vi "Servo.vi"() -> ()   [LabVIEW 2013]
doc: "This example shows how to set and read the angle of a servo."
uses:
  <vilib>/Rock Robotics/SystemInterfaces/DIO/FPGA_DIOPWMChannel.ctl
  <vilib>/Rock Robotics/SystemInterfaces/Typedef/FPGA_TypedefDigitalModule.ctl
panel:
  in  "DesiredAngle":i32
  in  "PWM Channel":T1=enum."PWM 6"
  out "Current Angle":u16(knob) scale=0.0..170.0
  in  "stop":bool
  # "1. Select the PWM channel for the servo.\n2. Press the run button\n3. Turn the Desired Angle to change the servo position\n4. The Current Angle is displayed in the dial\n5. Press STOP to end the program"
  # "Wiring Diagram for Digital Sidecar connected to an NI 9403"
  # "power jumper required for servo"
  # "The black wire should go into ground (-).\nThe red wire should go to power (PWR)\nThe white or yellow wire should go to signal (SIG)"
  # "PWR"
  # "SIG"
  # "(-)"
  # "+V"
  # "10"
  # "9"
  # "8"
  # "7"
  # "6"
  # "5"
  # "4"
  # "3"
  # "2"
  # "1"
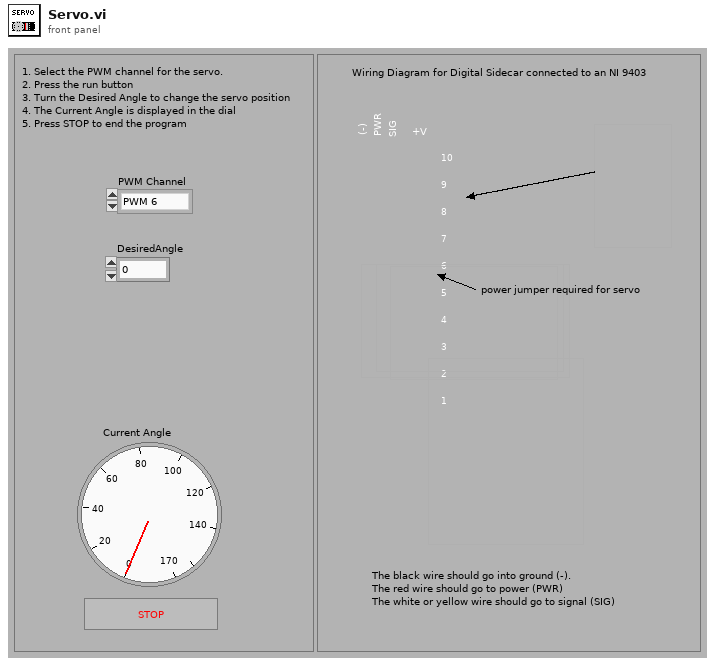
[diagram p1: front panel]
types:
  T1 = typedef "FPGA_DIOPWMChannel.ctl" = enum8{"PWM 1", "PWM 2", "PWM 3", "PWM 4", "PWM 5", "PWM 6", "PWM 7", "PWM 8", "PWM 9", "PWM 10", "Invalid"}
  T2 = typedef "FPGA_TypedefDigitalModule.ctl" = enum16{"Digital Module 1", "Digital Module 2"}
  T3 = typedef "WPI_ServoDeviceRef.ctl" = cluster{"DeviceStatus":errorcluster, "Digital Module":T2, "PWM Channel":T1, "DeadBand":T4}
  T4 = typedef "WPI_PWMDeadband.ctl" = cluster{"Name":string, "maxPositivePwm":i32, "minPositivePwm":i32, "centerPwm":i32, "maxNegativePwm":i32, "minNegativePwm":i32, "angularRange":u16}
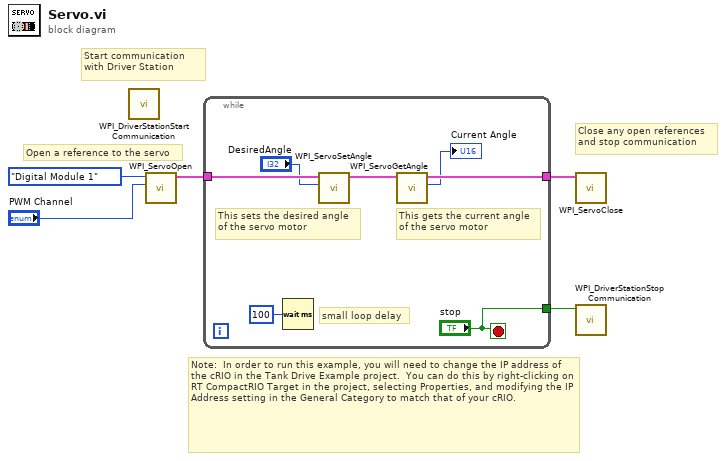
[diagram p0: block diagram]
diagram:
  # "Note:  In order to run this example, you will need to change the IP address of the cRIO in the Tank Drive Example project.  You can do this by right-clicking on RT CompactRIO Target in the project, selecting Properties, and modifying the IP Address setting in the General Category to match that of your cRIO."
  # "Close any open references\nand stop communication"
  # "Start communication with Driver Station"
  # "Open a reference to the servo"
  n1 = call <vilib>:"WPI_DriverStationStart Communication.vi"() -> ()  [unwired: 1 in, 11 out]
  n2 = call <vilib>:"WPI_ServoOpen.vi"("PWM Channel"="PWM Channel", "Digital Module (Module 1)"=FPGA_TypedefDigitalModule."Digital Module 1" ("DIO Module (Slot 4)")) -> ("ServoDeviceRef"=w5:T3)  [unwired: 2 in, 7 out]
  n3 = while {
    tunnel: w5 -> [w12]
    tunnel: [w10] -> w4
    tunnel: ["stop"] -> w1
    stop <- "stop" stop-if-true
    # "small loop delay"
    # "This gets the current angle\nof the servo motor"
    # "This sets the desired angle \nof the servo motor"
    n4 = Wait (ms)(milliseconds to wait=u32 100) -> ()  [unwired: 1 out]
    n5 = call <vilib>:"WPI_ServoSetAngle.vi"("Angle"="DesiredAngle", "ServoDeviceRef"=w12) -> ("ServoDeviceRef"=w11:T3)  [unwired: 1 in, 8 out]
    n6 = call <vilib>:"WPI_ServoGetAngle.vi"("ServoDeviceRef"=w11) -> ("ServoDeviceRef"=w10:T3, "Angle"=→"Current Angle":u16)  [unwired: 1 in, 7 out]
  }
  n7 = call <vilib>:"WPI_ServoClose.vi"("MotorControlDevRef"=w4) -> ()  [unwired: 1 in, 10 out]
  n8 = call <vilib>:"WPI_DriverStationStop Communication.vi"("StopCommunication"=w1) -> ()  [unwired: 1 in, 10 out]
